vi "Send UNSUBSCRIBE.vi"(8 "error in (no error)":errorcluster, 9 "Message loop data (in)":T1, 10 "Unsubscribe Request Data":T12, 11 "WAMP Client in":refnum<class "WAMP Client.lvclass">) -> (0 "error out":errorcluster, 1 "Message loop data (out)":T1, 3 "WAMP Client out":refnum<class "WAMP Client.lvclass">)   [LabVIEW 2020, in "wamplv.lvlib" / "WAMP Client.lvclass"]
uses:
  WAMP Client.lvclass
  WAMP Client.lvclass/WAMP Client.ctl
  API/TypeDefs/WAMP error.ctl
  API/TypeDefs/Combined error.ctl
  TypeDef/UNSUBSCRIBE Result.ctl
  342dd7b2-ead0-4019-b1f6-bfda333e20ae.vi
  TypeDef/EVENT payload.ctl
  TypeDef/UNSUBSCRIBE Request Data.ctl
  TypeDef/Unsubscribe Requests Map.ctl
  TypeDef/Subscription Details.ctl
  TypeDef/Subscriptions Map.ctl
  TypeDef/Success or error.ctl
  TypeDef/REGISTER Request Data.ctl
  TypeDef/PUBLISH Request Data.ctl
  TypeDef/Publish Requests Map.ctl
  TypeDef/Endpoint Data.ctl
  TypeDef/CALL Request Map.ctl
  TypeDef/Subscribe Result.ctl
  TypeDef/SUBSCRIBE Request Data.ctl
  TypeDef/SUBSCRIBE Requests Map.ctl
  TypeDef/Message Loop Data.ctl
  TypeDef/Unregister request.ctl
  TypeDef/Unregister requests map.ctl
  TypeDef/PUBLISH result.ctl
  Private/Requests/ICallRequest/ICallRequest.lvclass
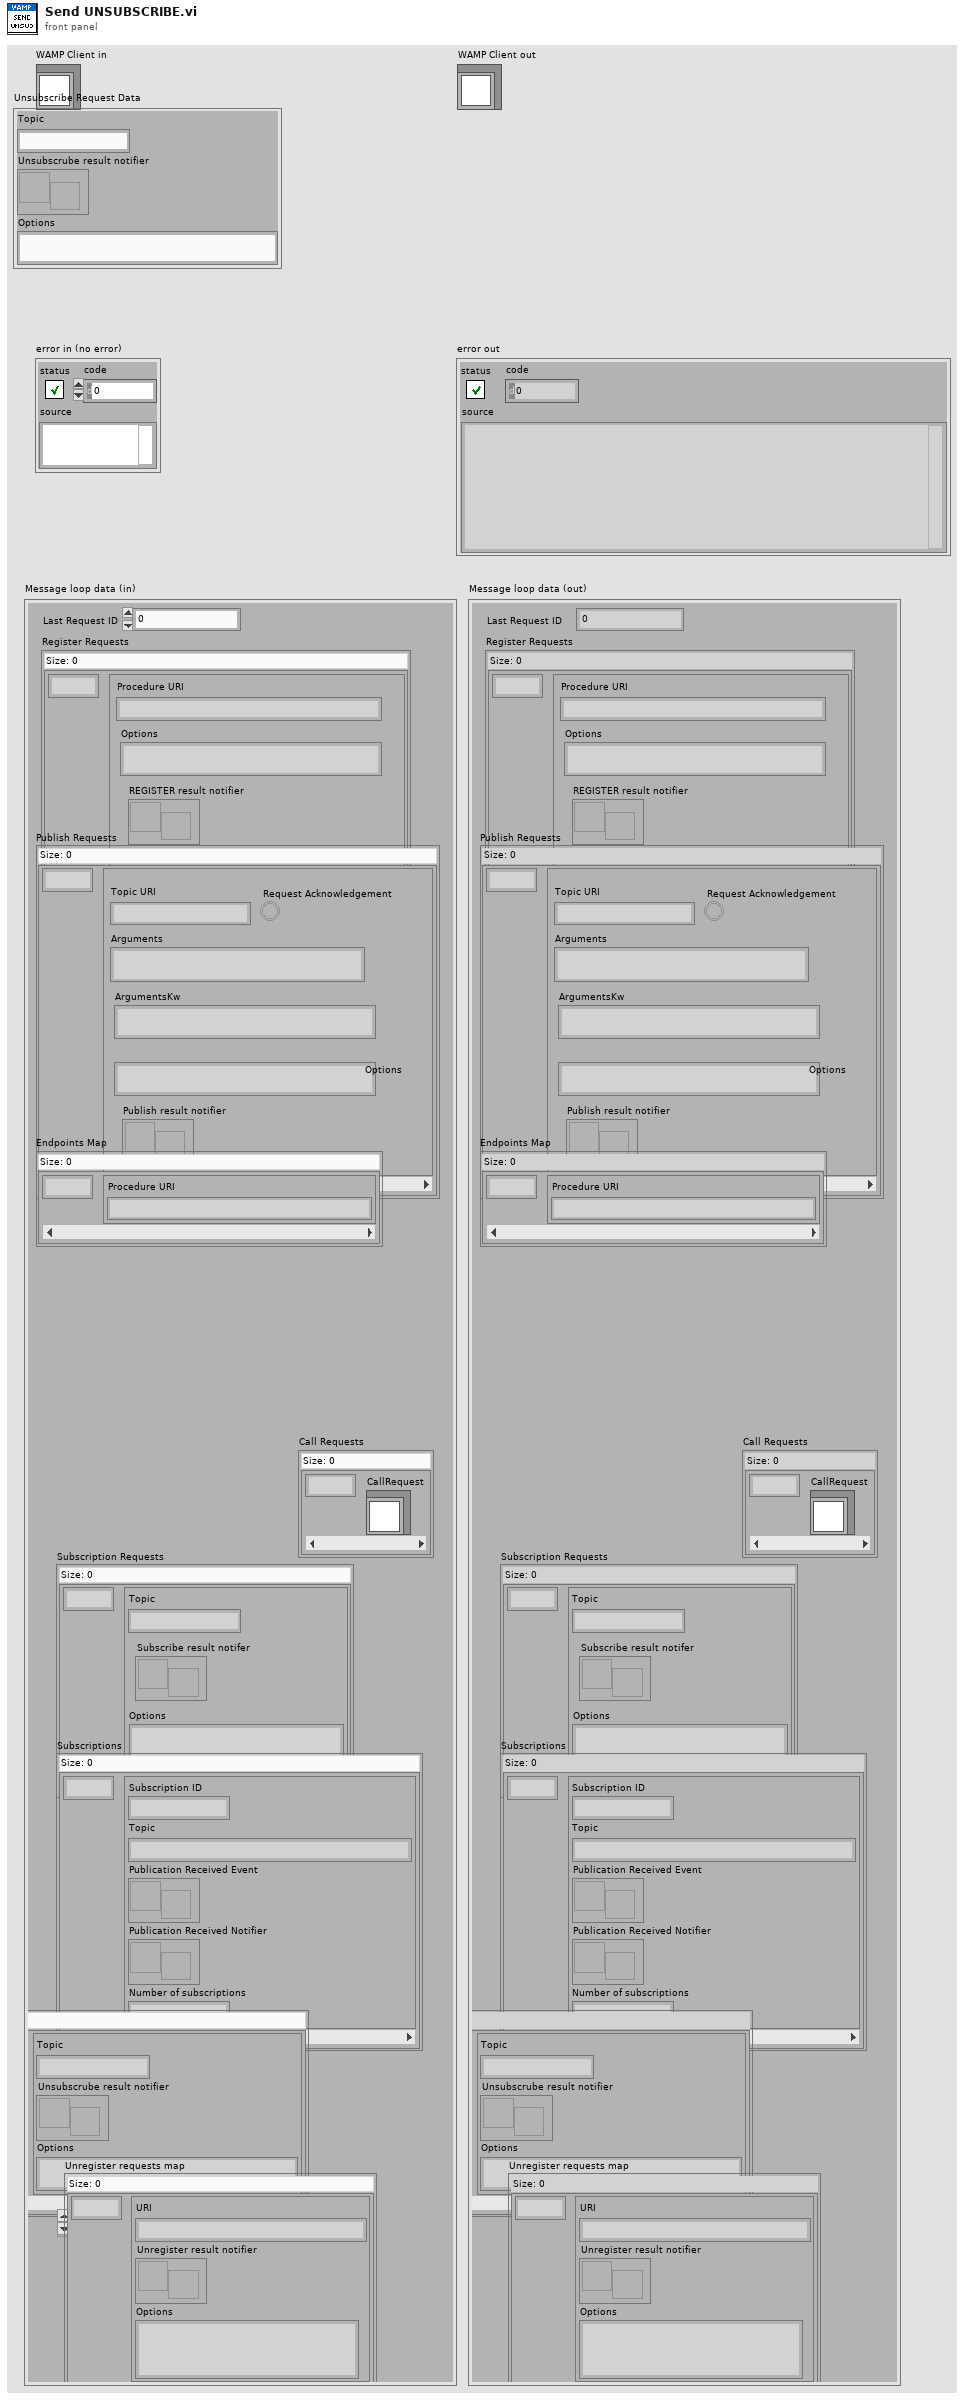
[diagram p1: front panel]
types:
  T1 = typedef "wamplv.lvlib/WAMP Client.lvclass/Message Loop Data.ctl" = cluster{"Last Request ID":u64, "Register Requests":map{u64, T2}, "Publish Requests":T3, "Endpoints Map":map{u64, T5}, "Call Requests":T6, "Subscription Requests":T7, "Subscriptions":T9, "Unsubscribe Requests":T11, "Random Request IDs":u64[], "Unregister requests map":T13}
  T2 = typedef "wamplv.lvlib/WAMP Client.lvclass/REGISTER Request Data.ctl" = cluster{"Procedure URI":string, "Options":string, "REGISTER result notifier":refnum<notifier>}
  T3 = typedef "wamplv.lvlib/WAMP Client.lvclass/Publish Requests Map.ctl" = map{u64, T4}
  T4 = typedef "wamplv.lvlib/WAMP Client.lvclass/PUBLISH Request Data.ctl" = cluster{"Topic URI":string, "Arguments":string, "ArgumentsKw":string, "Request Acknowledgement":bool, "Options":string, "Publish result notifier":refnum<notifier>}
  T5 = typedef "wamplv.lvlib/WAMP Client.lvclass/Endpoint Data.ctl" = cluster{"Procedure URI":string}
  T6 = typedef "wamplv.lvlib/WAMP Client.lvclass/CALL Request Map.ctl" = map{u64, refnum<class "ICallRequest.lvclass">}
  T7 = typedef "wamplv.lvlib/WAMP Client.lvclass/SUBSCRIBE Requests Map.ctl" = map{u64, T8}
  T8 = typedef "wamplv.lvlib/WAMP Client.lvclass/SUBSCRIBE Request Data.ctl" = cluster{"Topic":string, "Subscribe result notifer":refnum<notifier>, "Options":string}
  T9 = typedef "wamplv.lvlib/WAMP Client.lvclass/Subscriptions Map.ctl" = map{u64, T10}
  T10 = typedef "wamplv.lvlib/WAMP Client.lvclass/Subscription Details.ctl" = cluster{"Subscription ID":u64, "Topic":string, "Publication Received Event":refnum<user-event>, "Publication Received Notifier":refnum<notifier>, "Number of subscriptions":u64}
  T11 = typedef "wamplv.lvlib/WAMP Client.lvclass/Unsubscribe Requests Map.ctl" = map{u64, T12}
  T12 = typedef "wamplv.lvlib/WAMP Client.lvclass/UNSUBSCRIBE Request Data.ctl" = cluster{"Topic":string, "Unsubscrube result notifier":refnum<notifier>, "Options":string}
  T13 = typedef "wamplv.lvlib/WAMP Client.lvclass/Unregister requests map.ctl" = map{u64, T14}
  T14 = typedef "wamplv.lvlib/WAMP Client.lvclass/Unregister request.ctl" = cluster{"URI":string, "Unregister result notifier":refnum<notifier>, "Options":string}
  T15 = typedef "wamplv.lvlib/WAMP Client.lvclass/UNSUBSCRIBE Result.ctl" = cluster{"Success?":bool, "Combined Error":T16}
  T16 = typedef "wamplv.lvlib/WAMP Client.lvclass/Combined error.ctl" = cluster{"Error?":bool, "WAMP Error":T17, "Error":errorcluster}
  T17 = typedef "wamplv.lvlib/WAMP Client.lvclass/WAMP error.ctl" = cluster{"Details":string, "ArgumentKw Payload":string, "Error?":bool, "Error URI":string, "Arguments Payload":string}
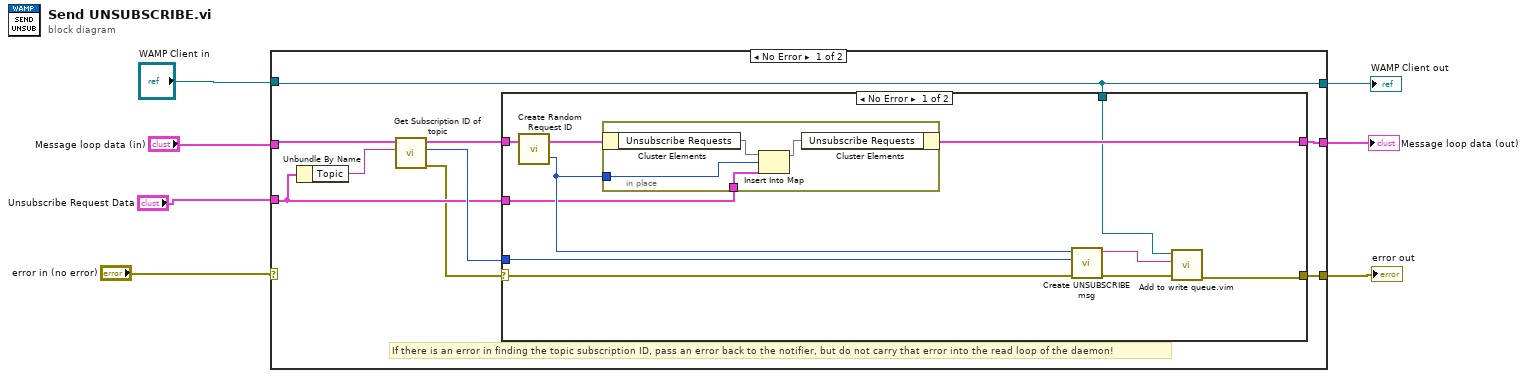
[diagram p0: block diagram]
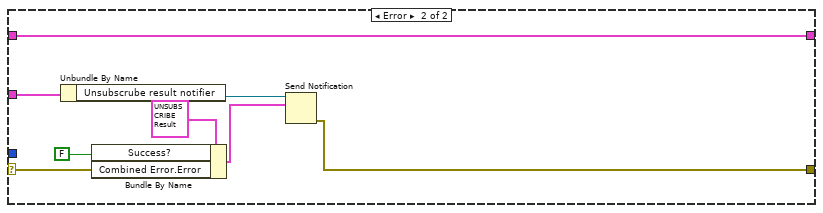
[diagram p2: hidden frame]
diagram:
  n1 = case shown="No Error" "error in (no error)" {
    selector: "error in (no error)" -> [_ w42]
    tunnel: [w15 w42] -> w6
    tunnel: [w16 w41] -> w4
    tunnel: "WAMP Client in" -> [w16 w41]
    tunnel: "Unsubscribe Request Data" -> [w12 _]
    tunnel: "Message loop data (in)" -> [w10 w40]
    tunnel: [w8 w40] -> w1
    frame No Error {
      # "If there is an error in finding the topic subscription ID, pass an error back to the notifier, but do not carry that error into the read loop of the daemon!"
      n2 = Unbundle By Name(w12) -> ("Topic"=w14:string)
      n3 = call "Get Subscription ID of topic.vi"("Topic"=w14, "Message loop data (in)"=w10) -> ("error out"=w9:errorcluster, "Subscription ID"=w13:u64, "Message loop data (out)"=w11:T1)  [unwired: 7 in]
      n4 = case shown="No Error" w9 {
        selector: w9 -> [w21 w35]
        tunnel: w16 -> [w19 _]
        tunnel: [w17 w32] -> w15
        tunnel: w13 -> [w26 _]
        tunnel: w12 -> [w25 w34]
        tunnel: w11 -> [w24 w39]
        tunnel: [w22 w39] -> w8
        frame No Error {
          n5 = call "Create Random Request ID.vi"("Message Loop Shift Register Data (in)"=w24) -> ("Generated Request ID"=w27:u64, "Message Loop Shift Register Data (out)"=w23:T1)  [unwired: 1 in]
          n6 = in-place "In Place Element Structure" {
            in-place-border: w27 -> [w31]
            in-place-border: w25 -> [w30]
            n7 = in-place-cluster #1(w23) -> ("Unsubscribe Requests"=w29:T11)
            n8 = Insert Into Map(map in=w29, key=w31, value=w30) -> (map out=w28:T11)  [unwired: 2 out]
            n9 = in-place-cluster #1("Unsubscribe Requests"=w28) -> (w22:T1)
          }
          n10 = call "Create UNSUBSCRIBE msg.vi"("error in (no error)"=w21, "Subscriiption ID"=w26, "Request ID"=w27) -> ("error out"=w20:errorcluster, "WAMP Message"=w18:string)  [unwired: 7 in]
          n11 = call "Add to write queue.vim"("error in (no error)"=w20, "Input"=w18, "WAMP Client in"=w19) -> ("error out"=w17:errorcluster)  [unwired: 8 in]
        }
        frame Error {
          n12 = Unbundle By Name(w34) -> ("Unsubscrube result notifier"=w38:refnum<notifier>)
          n13 = Bundle By Name(cluster=T15 {"Success?"=FALSE, "Combined Error"={"Error?"=FALSE, "WAMP Error"={"Details"="", "ArgumentKw Payload"="{}", "Error?"=FALSE, "Error URI"="", "Arguments Payload"=""}, "Error"={"status"=FALSE, "code"=0, "source"=""}}} ("Unsubcsribe Result"), "Success?"=FALSE, "Combined Error.Error"=w35) -> (w33:T15)
          n14 = Send Notification(notification=w33, notifier=w38) -> (error out=w32:errorcluster)  [unwired: 1 in, 1 out]
        }
      }
    }
    frame Error {
    }
  }
  "error out" <- w6
  "WAMP Client out" <- w4
  "Message loop data (out)" <- w1
